vi "Run.vi"(8 "error in (no error)":errorcluster, 11 "C37.118 Sim in":refnum<class "C37.118 Sim.lvclass">) -> (0 "error out":errorcluster, 1 "DataValid":bool, 2 "clSensorData":T1, 3 "C37.118 Sim out":refnum<class "C37.118 Sim.lvclass">)   [LabVIEW 2018, in "SensorPlugins.lvlib" / "C37.118 Sim.lvclass"]
uses:
  C37.118 Sim.lvclass
  C:/Users/ico/Documents/Projects/NistPluggableModules/Sensor/SensorPlugins/PmuBaseClass/PmuBase.lvclass
  SensorShared/clSensorData.ctl
  PmuBaseClass/PmuBase.lvclass/PmuBase.ctl
  C37.118 Sim.lvclass/C37.118 Sim.ctl
  PmuBaseClass/Accessors/Read PmuDataArray.vi
  Accessors/Read Reporting period.vi
  PmuBaseClass/Accessors/Write PmuDataArray.vi
  SensorShared/SensorShared.lvlib
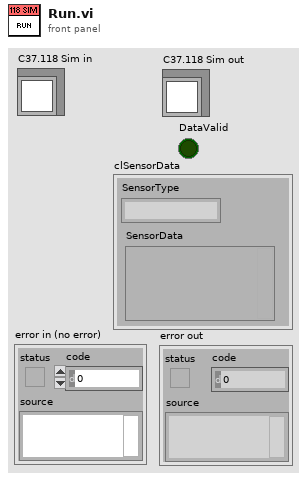
[diagram p1: front panel]
types:
  T1 = typedef "SensorShared.lvlib/clSensorData.ctl" = cluster{"SensorType":string, "SensorData":variant}
  T2 = typedef "SensorPlugins.lvlib/PmuBase.lvclass/PmuData.ctl" = cluster{"Timestamp":dbl, "Synx":cdb[], "Freq":dbl, "ROCOF":dbl, "ID":i16}
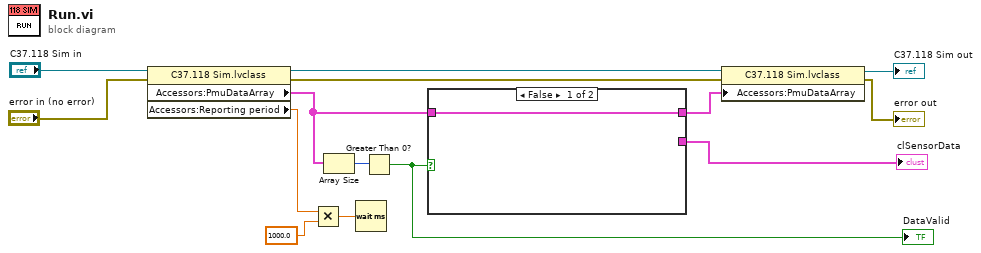
[diagram p0: block diagram]
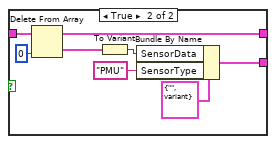
[diagram p2: hidden frame]
diagram:
  n1 = property class="C37.118 Sim.lvclass"(reference="C37.118 Sim in", error in="error in (no error)") -> (reference out=w11:refnum<class "C37.118 Sim.lvclass">, error out=w10:errorcluster, "Accessors:PmuDataArray"=w3:T2[], "Accessors:Reporting period"=w5:dbl)
  n2 = Multiply(x=w5, y=1000.0) -> (x*y=w7:dbl)
  n3 = Array Size(array=w3) -> (size(s)=w2:i32)
  n4 = Wait (ms)(milliseconds to wait=w7) -> ()  [unwired: 1 out]
  n5 = Greater Than 0?(x=w2) -> (x > 0?=w1:bool)
  "DataValid" <- w1
  n6 = case shown="False" w1 {
    tunnel: [_ w23] -> w8
    tunnel: [w15 w18] -> w4
    tunnel: w3 -> [w15 w16]
    frame False {
    }
    frame True {
      n7 = Delete From Array(array=w16, index=0) -> (deleted portion=w19:T2, array with subset deleted=w18:T2[])  [unwired: 1 in]
      n8 = To Variant(anything=w19) -> (Variant=w21:variant)
      n9 = Bundle By Name(cluster=T1 {"SensorType"="", "SensorData"=variant} ("clSensorData"), "SensorData"=w21, "SensorType"="PMU") -> (w23:T1)
    }
  }
  "clSensorData" <- w8
  n10 = property class="C37.118 Sim.lvclass"(reference=w11, error in=w10, "Accessors:PmuDataArray"=w4) -> (reference out=→"C37.118 Sim out":refnum<class "C37.118 Sim.lvclass">, error out=→"error out":errorcluster)
